vi "Set Shifter.vi"(8 "error in (no error)":errorcluster, 10 "Override?":bool, 11 "Gear (F = Low Gear)":bool) -> (0 "error out":errorcluster)   [LabVIEW 2015]
uses:
  <vilib>/Rock Robotics/WPI/Solenoid/WPI_SolenoidValue.ctl
  <vilib>/Rock Robotics/WPI/Power/WPI_Power Get 5Volt Rail Voltage and Current.vi
  <vilib>/Rock Robotics/WPI/Solenoid/WPI_SolenoidSetEnum.vi
  <vilib>/Rock Robotics/Network Tables/NT Write String.vi
panel:
  out "Pressure":dbl(graph)
  in  "Max Pressure":dbl=40.0
  # "<--~40psi"
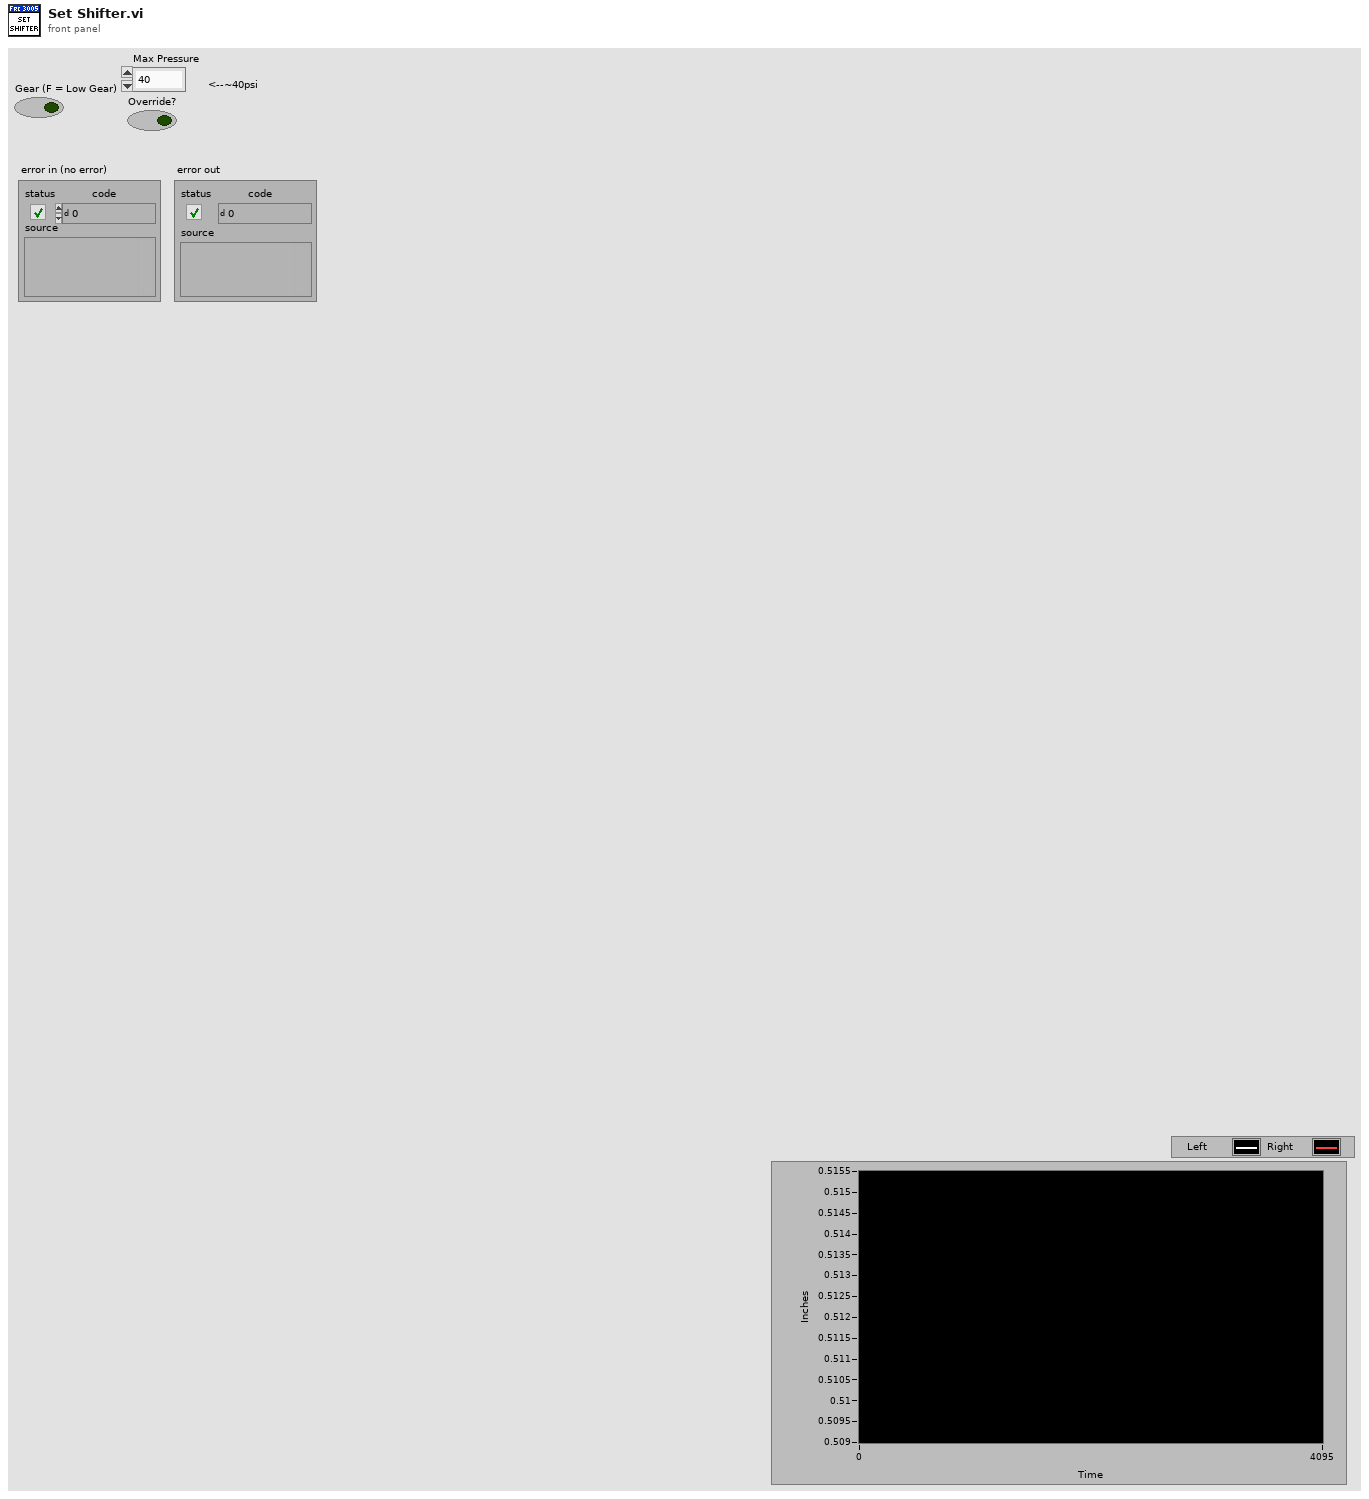
[diagram p1: front panel]
types:
  T1 = typedef "WPI_AnalogChannelDevRef.ctl" = cluster{"DevStatus":errorcluster, "Analog Channel":T2}
  T2 = typedef "FPGA_AIChannel.ctl" = enum8{"AI 0", "AI 1", "AI 2", "AI 3", "AI MXP 0", "AI MXP 1", "AI MXP 2", "AI MXP 3", "Invalid"}
  T3 = typedef "WPI_SolenoidValue.ctl" = enum16{"Off", "On", "Forward", "Reverse"}
  T4 = typedef "WPI_SolenoidDevRef.ctl" = cluster{"DevStatus":errorcluster, "Pneumatics Control Module":u8, "Forward Solenoid Channel":T5, "Reverse Solenoid Channel":T5}
  T5 = typedef "WPI_SolenoidChannel.ctl" = enum8{"Solenoid 0", "Solenoid 1", "Solenoid 2", "Solenoid 3", "Solenoid 4", "Solenoid 5", "Solenoid 6", "Solenoid 7", "Invalid"}
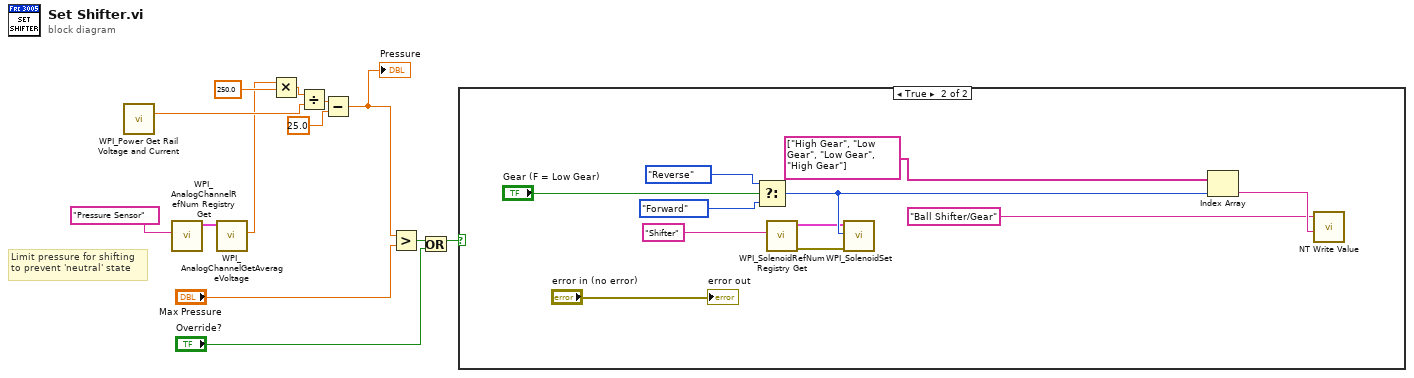
[diagram p0: block diagram]
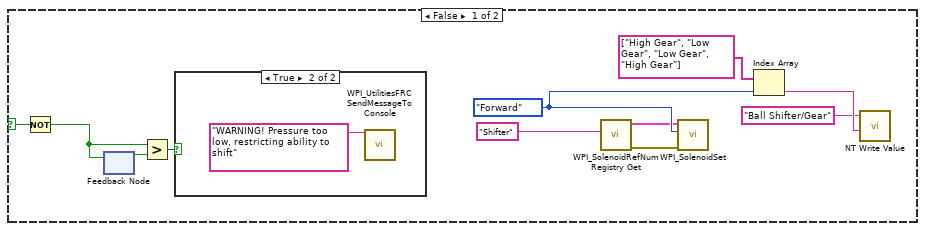
[diagram p2: hidden frame]
diagram:
  # "Limit pressure for shifting\nto prevent 'neutral' state"
  n1 = call-poly <vilib>:"WPI_Power Get Rail Voltage and Current.vi"() -> ("5 volt rail voltage (V)"=w6:dbl)  [unwired: 13 in, 2 out]
  n2 = call <vilib>:"WPI_AnalogChannelRefNum Registry Get.vi"("refnum name"="Pressure Sensor") -> ("AIDeviceRef"=w12:T1)  [unwired: 9 in, 1 out]
  n3 = call <vilib>:"WPI_AnalogChannelGetAverageVoltage.vi"("AIDeviceRef"=w12) -> ("Voltage"=w2:dbl)  [unwired: 8 in, 2 out]
  n4 = Multiply(x=w2, y=250.0) -> (x*y=w3:dbl)
  n5 = Divide(x=w3, y=w6) -> (x/y=w4:dbl)
  n6 = Subtract(x=w4, y=25.0) -> (x-y=w1:dbl)
  "Pressure" <- w1
  n7 = Greater?(x=w1, y="Max Pressure") -> (0:w11:bool)
  n8 = Or(x=w11, y="Override?") -> (x .or. y?=w9:bool)
  n9 = case shown="True" w9 {
    selector: w9 -> [w24 _]
    frame False {
      w19 = WPI_SolenoidValue."Forward" ("Value")
      n10 = Not(x=w24) -> (.not. x?=w22:bool)
      n11 = feedback-in #1(w22) -> ()
      n12 = feedback #1() -> (w23:bool)  [unwired: 1 in]
      n13 = Greater?(x=w22, y=w23) -> (0:w21:bool)
      n14 = case shown="True" w21 {
        frame False {
        }
        frame True {
          n15 = call <vilib>:"WPI_UtilitiesFRC SendMessageToConsole.vi"("Message"="WARNING! Pressure too low, restricting ability to shift") -> ()  [unwired: 14 in, 1 out]
        }
      }
      n16 = call <vilib>:"WPI_SolenoidRefNum Registry Get.vi"("refnum name"="Shifter") -> ("error out"=w16:errorcluster, "SolenoidDevRef"=w15:T4)  [unwired: 9 in]
      n17 = call-poly <vilib>:"WPI_SolenoidSet.vi"("error in (no error)"=w16, "Value"=w19, "SolenoidDevRef"=w15) -> ()  [unwired: 7 in, 2 out]
      n18 = Index Array(array=string[] ["High Gear", "Low Gear", "Low Gear", "High Gear"], index=w19) -> (element=w20:string)
      n19 = call-poly <vilib>:"NT Write Value.vi"("String"=w20, "Name"="Ball Shifter/Gear") -> ()  [unwired: 9 in, 1 out]
    }
    frame True {
      n20 = Select(t=WPI_SolenoidValue."Reverse" ("Value"), s="Gear (F = Low Gear)", f=WPI_SolenoidValue."Forward" ("Value")) -> (s? t:f=w35:T3)
      n21 = call <vilib>:"WPI_SolenoidRefNum Registry Get.vi"("refnum name"="Shifter") -> ("error out"=w29:errorcluster, "SolenoidDevRef"=w28:T4)  [unwired: 9 in]
      n22 = call-poly <vilib>:"WPI_SolenoidSet.vi"("error in (no error)"=w29, "Value"=w35, "SolenoidDevRef"=w28) -> ()  [unwired: 7 in, 2 out]
      n23 = Index Array(array=string[] ["High Gear", "Low Gear", "Low Gear", "High Gear"], index=w35) -> (element=w36:string)
      n24 = call-poly <vilib>:"NT Write Value.vi"("String"=w36, "Name"="Ball Shifter/Gear") -> ()  [unwired: 9 in, 1 out]
      "error out" <- "error in (no error)"
    }
  }
